vi "niRFUtil WFM Apply Headroom.vi"(2 "Headroom, dB (-1 = Auto)":T1=-1.0 format="%.1f", 3 "Complex Signal In":T2 {"y" format="%.2f"; "dx" format="%^.2e"; "x0" format="%^.2e"}) -> (0 "Actual Headroom, dB":T1 format="%.1f", 1 "Complex Signal Out":T2 {"y" format="%.2f"; "dx" format="%^.2e"; "x0" format="%^.2e"})   [LabVIEW 2015, in "niRFUtil.lvlib"]
doc: "(c) Copyright 2006, National Instruments, Inc. This VI may not be duplicated, sold, or distributed without written consent from National Instruments."
uses:
  niRFUtil.lvlib
  Includes/niRFUtil INC Complex Waveform.ctl
  Includes/niRFUtil INC Complex Array.ctl
  Includes/niRFUtil INC Headroom.ctl
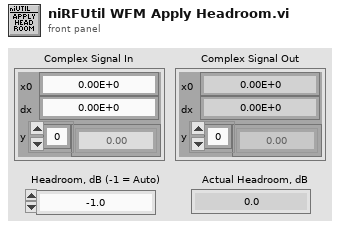
[diagram p1: front panel]
types:
  T1 = typedef "niRFUtil.lvlib/niRFUtil INC Headroom.ctl" = sgl
  T2 = typedef "niRFUtil.lvlib/niRFUtil INC Complex Waveform.ctl" = cluster{"x0":dbl, "dx":dbl, "y":T3}
  T3 = typedef "niRFUtil.lvlib/niRFUtil INC Complex Array.ctl" = csg[]
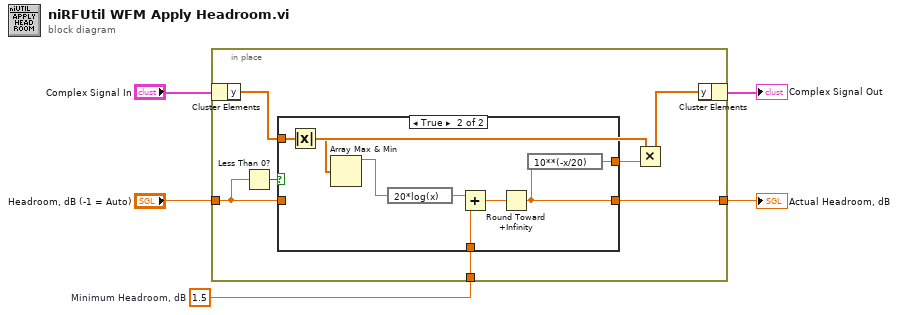
[diagram p0: block diagram]
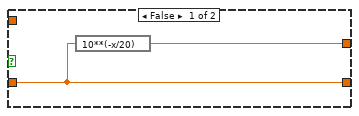
[diagram p2: hidden frame]
diagram:
  w1 = T1 1.5  # Minimum Headroom, dB
  n1 = in-place {
    in-place-border: "Headroom, dB (-1 = Auto)" -> [w6]
    in-place-border: [w11] -> w3
    in-place-border: w1 -> [w8]
    n2 = in-place-cluster #1("Complex Signal In") -> ("y"=w10:T3)
    n3 = Less Than 0?(x=w6) -> (x < 0?=w7:bool)
    n4 = case shown="True" w7 {
      tunnel: [w14 w19] -> w12
      tunnel: w6 -> [w13 _]
      tunnel: w10 -> [_ w22]
      tunnel: [w13 w20] -> w11
      tunnel: w8 -> [_ w17]
      frame False {
        n5 = expression code="10**(-x/20)"(w13) -> (w14:T1)
      }
      frame True {
        n6 = Absolute Value(x=w22) -> (abs(x)=w21:sgl[])
        n7 = Array Max & Min(array=w21) -> (max value=w15:sgl)  [unwired: 3 out]
        n8 = expression code="20*log(x)"(w15) -> (w18:sgl)
        n9 = Add(x=w18, y=w17) -> (x+y=w16:T1)
        n10 = Round Toward +Infinity(x=w16) -> (ceil(x): smallest int >= x=w20:T1)
        n11 = expression code="10**(-x/20)"(w20) -> (w19:T1)
      }
    }
    n12 = Multiply(x=w10, y=w12) -> (x*y=w9:T3)
    n13 = in-place-cluster #1("y"=w9) -> (→"Complex Signal Out":T2)
  }
  "Actual Headroom, dB" <- w3
